vi "Key Information.vi"(7 "Section Name":string, 8 "error in (no error)":errorcluster, 10 "Key Name":string, 11 "Config in":refnum<class "LabVIEW-Config.lvclass">) -> (0 "error out":errorcluster, 2 "Key Information":T1[](array[typedef]), 3 "Config out":refnum<class "LabVIEW-Config.lvclass">)   [LabVIEW 2017, in "LabVIEW-Config.lvlib" / "LabVIEW-Config.lvclass"]
uses:
  LabVIEW-Config.lvclass
  KeyInfo.ctl
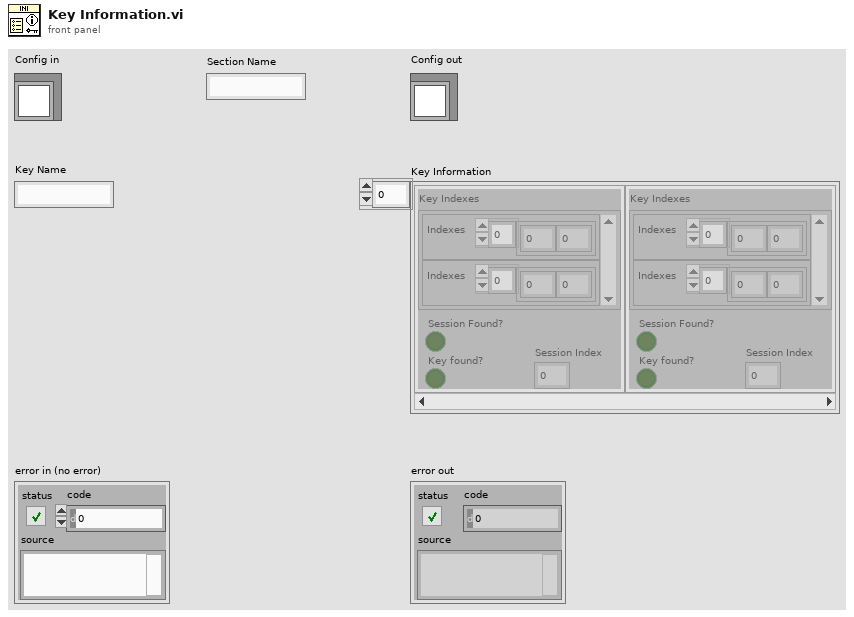
[diagram p1: front panel]
types:
  T1 = typedef "LabVIEW-Config.lvlib/LabVIEW-Config.lvclass/KeyInfo.ctl" = cluster{"Key Indexes":cluster{"Indexes":i32[]}[], "Session Found?":bool, "Key found?":bool, "Session Index":i32}
  T2 = typedef "LabVIEW-Config.lvlib/LabVIEW-Config.lvclass/SessionInfo.ctl" = cluster{"Session Indexes":i32[]}
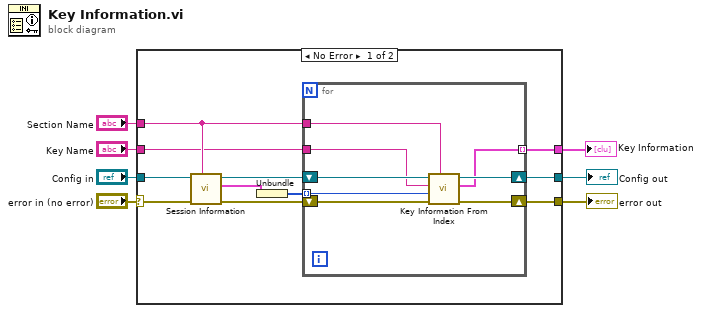
[diagram p0: block diagram]
diagram:
  n1 = case shown="No Error" "error in (no error)" {
    selector: "error in (no error)" -> [w10 w28]
    tunnel: "Config in" -> [w18 w27]
    tunnel: [w9 w28] -> w6
    tunnel: [w16 w27] -> w4
    tunnel: "Section Name" -> [w15 _]
    tunnel: "Key Name" -> [w12 _]
    tunnel: [w8 _] -> w1
    frame No Error {
      n2 = call "Session Information.vi"("Section Name"=w15, "error in (no error)"=w10, "Config in"=w18) -> ("error out"=w11:errorcluster, "Session Information"=w14:T2, "Config out"=w17:refnum<class "LabVIEW-Config.lvclass">)  [unwired: 6 in]
      n3 = Unbundle(w14) -> ("Session Indexes"=w13:i32[])
      n4 = for {
        tunnel: w15 -> [w24]
        tunnel: w13 -> [w23] mode=indexing
        tunnel: w12 -> [w22]
        shift-right: [w25] -> w16
        shift-left: w17 -> [w26]
        shift-right: [w20] -> w9
        shift-left: w11 -> [w21]
        tunnel: [w19] -> w8 mode=indexing
        n5 = call "Key Information From Index.vi"("Section Name"=w24, "error in (no error)"=w21, "Start"=w23, "Key Name"=w22, "Config in"=w26) -> ("error out"=w20:errorcluster, "Key Information"=w19:T1, "Config out"=w25:refnum<class "LabVIEW-Config.lvclass">)  [unwired: 4 in]
      }
    }
    frame Error {
    }
  }
  "error out" <- w6
  "Config out" <- w4
  "Key Information" <- w1
